vi "Read Drive Operation.vi"(8 "Command Info":T4) -> (0 "Command Info":T4, 1 "SubSystem Data":T1, 2 "Command Timing":cluster{"Start Time (ms)":u32, "Iterations":i32})   [LabVIEW 2020]
doc: "Returns the details about the currently executing command."
uses:
  Implementation/Drive Operations.ctl
  Implementation/Drive Setpoints.ctl
  Implementation/Robot Velocities.ctl
  <vilib>/Rock Robotics/WPI/Framework/Completion Status.ctl
  <vilib>/Rock Robotics/WPI/Framework/Completion Notifier.ctl
  <vilib>/Rock Robotics/WPI/Framework/Command Status Info.ctl
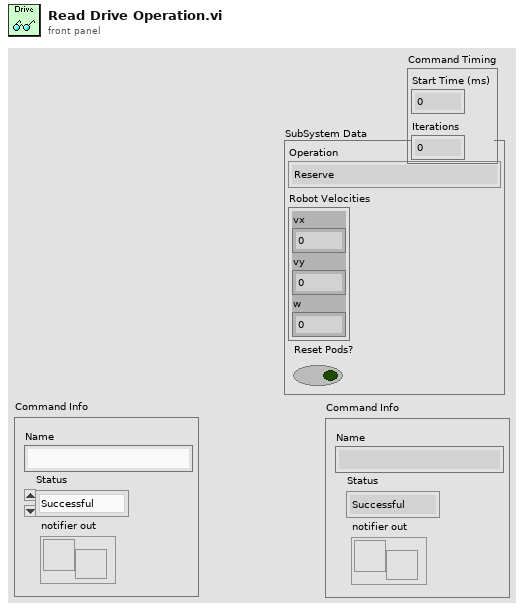
[diagram p1: front panel]
types:
  T1 = typedef "Drive Setpoints.ctl" = cluster{"Operation":T2, "Robot Velocities":T3, "Reset Pods?":bool}
  T2 = typedef "Drive Operations.ctl" = enum16{"Reserve", "Read Current", "Immediate", "Calibrate"}
  T3 = typedef "Robot Velocities.ctl" = cluster{"vx":dbl, "vy":dbl, "w":dbl}
  T4 = typedef "Command Status Info.ctl" = cluster{"Name":string, "Status":T5, "notifier out":T6}
  T5 = typedef "Completion Status.ctl" = enum16{"Successful", "Aborted", "Incomplete"}
  T6 = typedef "Completion Notifier.ctl" = refnum<notifier>
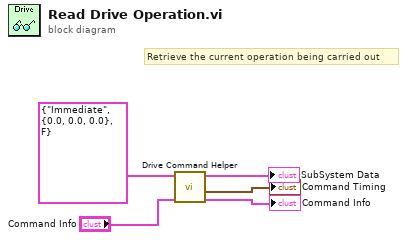
[diagram p0: block diagram]
diagram:
  # "Retrieve the current operation being carried out"
  n1 = call "Drive Command Helper.vi"("Command Info In"="Command Info", "SubSystem Data"=T1 {"Operation"=enum."Immediate", "Robot Velocities"={"vx"=0.0, "vy"=0.0, "w"=0.0}, "Reset Pods?"=FALSE}) -> ("Command Info Out"=→"Command Info":T4, "Command Timing"=→"Command Timing":cluster{"Start Time (ms)":u32, "Iterations":i32}, "SubSystem Data"=→"SubSystem Data":T1)  [unwired: 7 in]
